vi "MAG_UI_Main_old.vi"() -> ()   [LabVIEW 2016]
doc: "Use this template to build a simple state machine design pattern. Each state executes code and determines which state to transition to."
uses:
  controls/MAG_UI_Data.ctl
  controls/MAG_UI_Command.ctl
  controls/MAG_Comms_State.ctl
  controls/Sensor_Data.ctl
  <vilib>/Math Plots/3D Math Plots/3D Surface/3D Surface XCtrl/3D Surface.xctl
  <vilib>/Math Plots/3D Math Plots/3D Surface/3D Surface Datatype/3D Surface Datatype.lvclass
  controls/MAG_UI_State.ctl
  controls/MAG_Display_State.ctl
  controls/MAG_UI_Comms_Config.ctl
  <vilib>/Math Plots/3D Math Plots/3D Surface/3D Surface Datatype/Public/Plot Helper (Matrix).vi
panel:
  in  "UI_Tab":enum32{"Display", "Config", "Debug"}(tab)
  out "Sensor Readings":dbl[][](array[numeric])=[[53.321, -3127.915, -23851.52], [-458.11, -296.645, -18895.36], [1342.037, -322.179, -20134.399999999998], [1022.111, -1906.789, -22302.72], [2748.66, -1244.407, -21063.68], [-84.112, -4542.048, -19824.64], [307.91, 878.67, -19824.64], [-4568.333, -4041.882, -21373.44], [-6.008, -325.183, -24161.28], [-1336.78, 741.988, -16417.28], [596.294, -402.536, -21373.44], [-4497.739, -1861.729, -15488.0], [-2729.134, -3046.807, -17966.079999999998], [-4886.757, -3190.248, -15488.0], [-5275.775, -1495.241, -18585.6], [-744.241, -4708.019, -20753.92], [-2035.961, 1997.66, -22612.48], [-624.081, -1578.602, -21373.44], [-5331.349, -177.987, -15797.76], [-5163.876, -1893.271, -17656.32], [-6317.412, 26.285, -17036.8], [-5709.853, -1238.3990000000001, -17346.559999999998], [-6253.577, -2501.581, -17346.559999999998], [-4917.548, 525.7, -19514.88], [4038.127, 854.638, -17656.32], [2519.605, -2692.335, -17346.559999999998], [422.062, -178.738, -27878.399999999998], [2497.826, 931.24, -16417.28], [2088.531, 18.024, -17656.32], [-2016.435, -340.954, -16107.52], [1248.162, -1542.554, -20444.16], [-2485.059, -2575.179, -20444.16], [-69.092, -449.098, -22612.48], [-2240.984, 1145.275, -17346.559999999998], [3456.102, 2005.17, -17346.559999999998], [-3088.112, 773.53, -17036.8], [-1416.386, 1058.91, -18585.6], [-1229.387, 273.364, -18895.36], [-4542.048, -1396.86, -18895.36], [-4826.677, -60.08, -16417.28], [1227.134, 4367.065, -21063.68], [1716.786, 2915.382, -20134.399999999998], [-1334.527, 4276.194, -21373.44], [-884.678, 2008.174, -17036.8], [-1700.264, 2225.964, -21063.68], [-1527.534, 1893.271, -18895.36], [-2355.136, 772.028, -17346.559999999998], [-4691.497, -1109.227, -23541.76], [1372.828, 0.0, -23851.52], [-2353.634, 566.254, -21373.44], [-4619.401, 7687.987, -16417.28], [-6183.734, 823.096, -17036.8], [-5976.458, -100.634, -20444.16], [-3851.128, -639.101, -16417.28], [-4383.587, -1360.812, -19205.12], [-3419.303, -80.357, -17966.079999999998], [-3107.638, 4759.838, -22922.239999999998], [-3023.526, 2978.466, -19824.64], [-2249.245, 102.136, -20134.399999999998], [-714.201, -5060.989, -28188.16], [-950.015, 5369.65, -25710.079999999998], [-5348.622, 5862.306, -22612.48], [-3420.054, 3359.223, -19824.64], [-5260.004, 1431.406, -24780.8]]
  in  "Zero":bool
  in  "Tab Control":enum32{"2D", "3D"}(tab)=enum."3D"
  out "Node Response":T1(graph)={"Node XYZ List[0]"=53.321, "Node XYZ List[1]"=-3127.915, "Node XYZ List[2]"=-23851.52}
  in  "Node":i32
  out "3D Surface":refnum<class "3D Plot Datatype.lvclass">[](xcontrol)
  in  "Comms Setting":enum32{"Serial", "Bluetooth"}(tab)
  in  "VISA resource name":refnum<visa-resource-name>="COM16"
  in  "Serial Settings":T2={"baud rate"=57600, "data bits"=8, "parity"=enum."None", "stop bits"=10, "flow control"=0} {"flow control" items=["None"=0, "XON/XOFF"=1, "RTS/CTS"=2, "DTR/DSR"=4]; "stop bits" items=["1.0"=10, "1.5"=15, "2.0"=20]; "data bits" min=5 max=8 step=1; "baud rate" items=["75"=75, "110"=110, "134"=134, "150"=150, "300"=300, "600"=600, "1200"=1200, "1800"=1800, "2400"=2400, "4800"=4800, "7200"=7200, "9600"=9600, "14400"=14400, "19200"=19200, "28800"=28800, "38400"=38400, "56000"=56000, "57600"=57600, "115200"=115200, "128000"=128000, "230400"=230400]}
  out "Comm State":T3
  out "notification":T5
  out "comms":i32=4022
  out "ui":i32=2010
  out "Bytes_In_Buffer":u32
  in  "Button_Disconnect":bool
  in  "Button_Initialise":bool
  in  "Button_Stream":bool
  out "Status":T6={"System Version"="", "Connected"=TRUE, "Active?"=FALSE, "Streaming"=TRUE, "Logging"=FALSE}
  in  "Button_Record":bool
  in  "Button_Sys_Check":bool
  in  "Button_Connect":bool
  in  "Button_Exit":bool
  # "MagBoard n64"
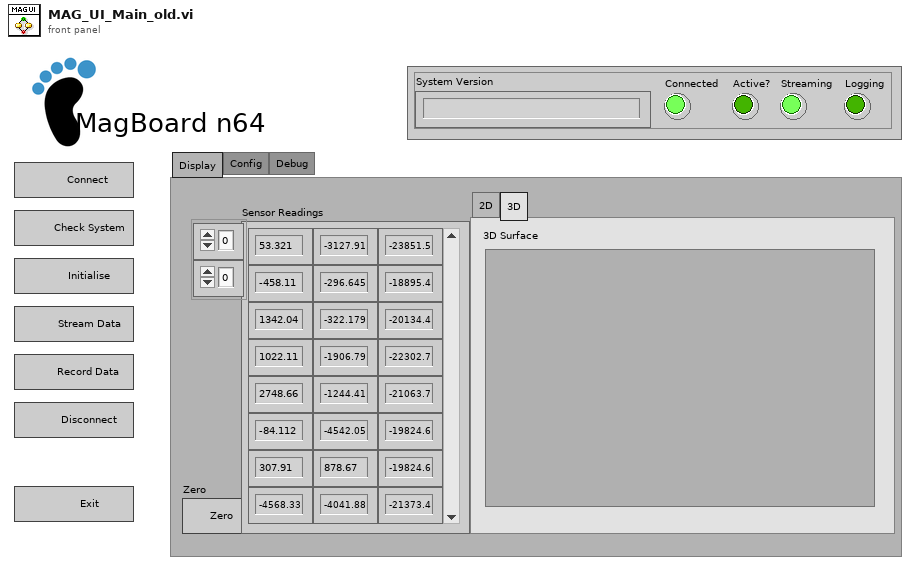
[diagram p1: front panel]
types:
  T1 = cluster{"Node XYZ List[0]":dbl, "Node XYZ List[1]":dbl, "Node XYZ List[2]":dbl}
  T2 = cluster{"baud rate":u32, "data bits":u16, "parity":enum16{"None", "Odd", "Even", "Mark", "Space"}, "stop bits":u16, "flow control":u16}
  T3 = typedef "MAG_UI_Command.ctl" = cluster{"Comms_States":T4, "Parameters":string, "Clear Buffer?":bool}
  T4 = typedef "MAG_Comms_State.ctl" = enum16{"Initialize", "Wait for Event", "Connect", "Send_Com", "Rcv_TXT", "Rcv_BIN", "Rcv_FILE", "Disconnect"}
  T5 = typedef "Sensor_Data.ctl" = cluster{"Time":u32, "Data":i16[]}
  T6 = typedef "MAG_UI_Data.ctl" = cluster{"System Version":string, "Connected":bool, "Active?":bool, "Streaming":bool, "Logging":bool}
  T7 = typedef "MAG_UI_Comms_Config.ctl" = cluster{enum16{"Serial", "Bluetooth"}, "Serial Refnum":refnum<visa-resource-name>}
  T8 = typedef "MAG_Display_State.ctl" = enum16{"Initialise", "Display", "Exit"}
  T9 = typedef "MAG_UI_State.ctl" = enum16{"Initialize", "Wait for Event", "Com_Connect", "Com_Init_Sys", "Com_Chk_Sys", "Com_Stream", "Com_Log", "Exit"}
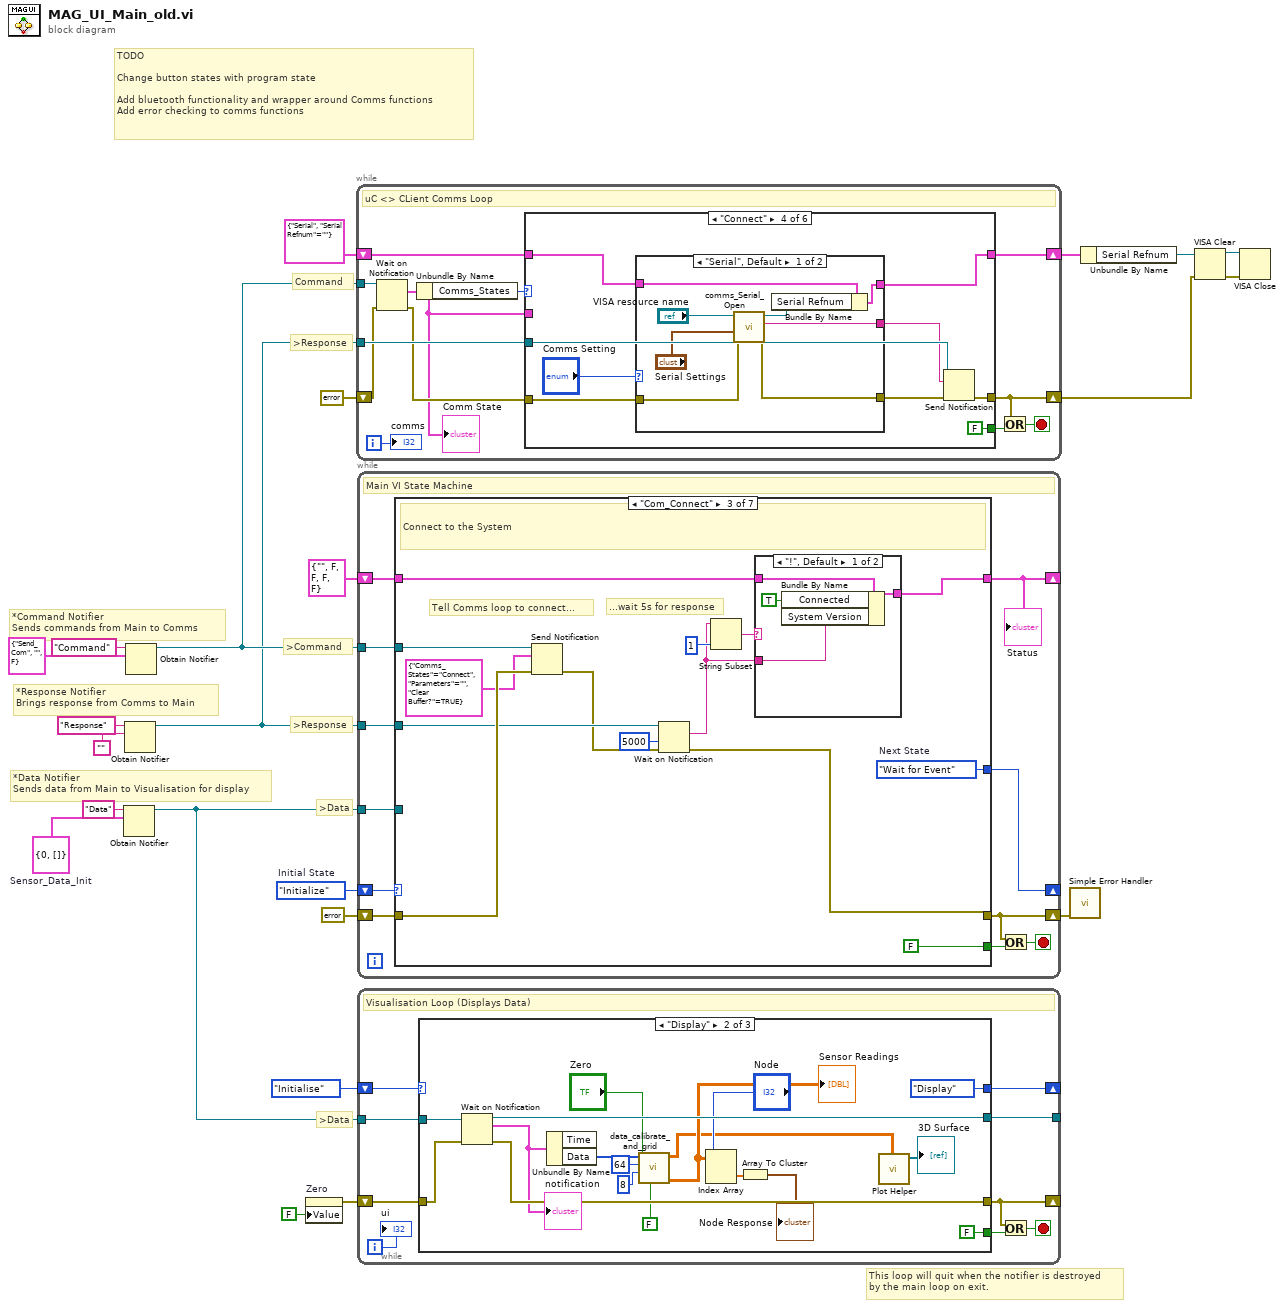
[diagram p0: block diagram]
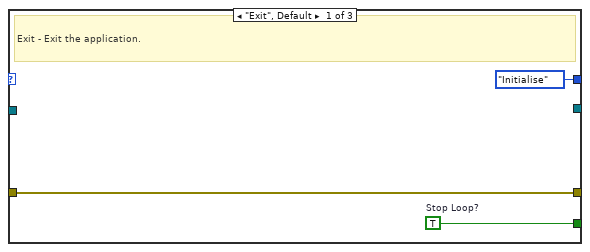
[diagram p2: hidden frame]
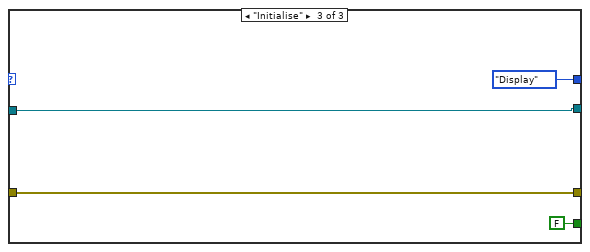
[diagram p3: hidden frame]
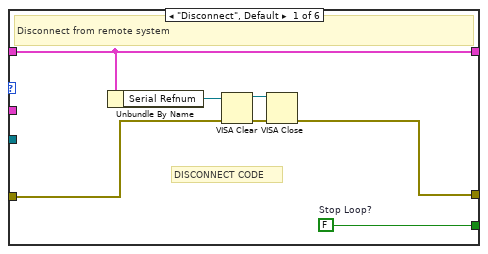
[diagram p4: hidden frame]
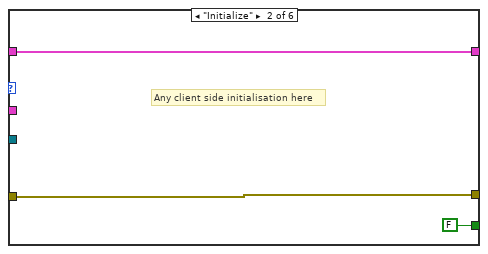
[diagram p5: hidden frame]
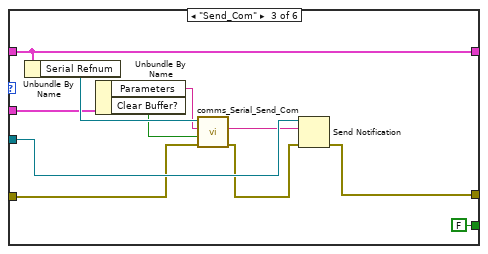
[diagram p6: hidden frame]
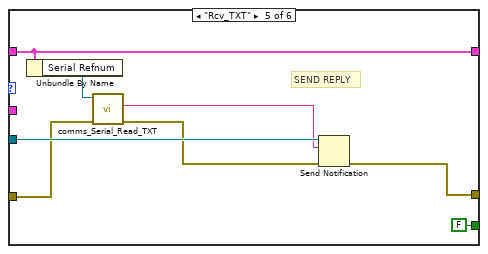
[diagram p8: hidden frame]
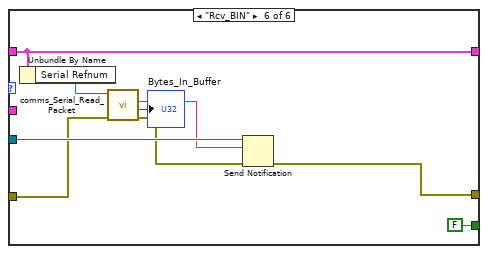
[diagram p9: hidden frame]
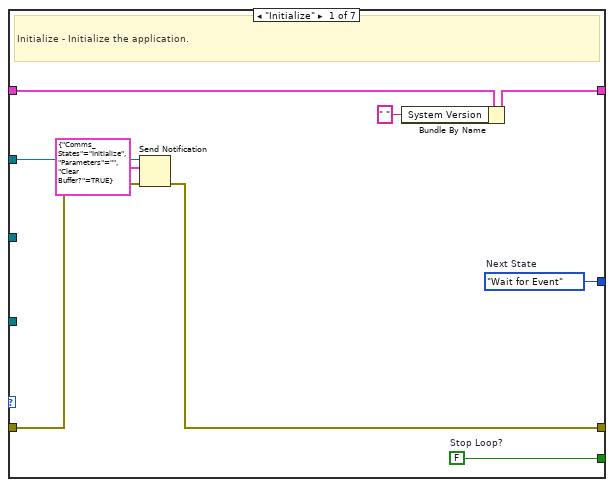
[diagram p10: hidden frame]
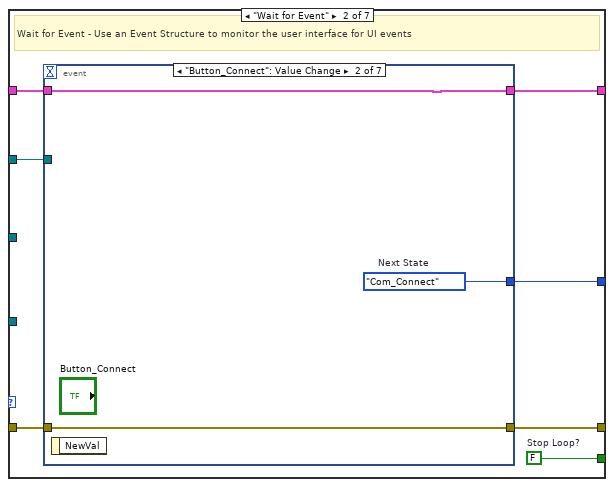
[diagram p11: hidden frame]
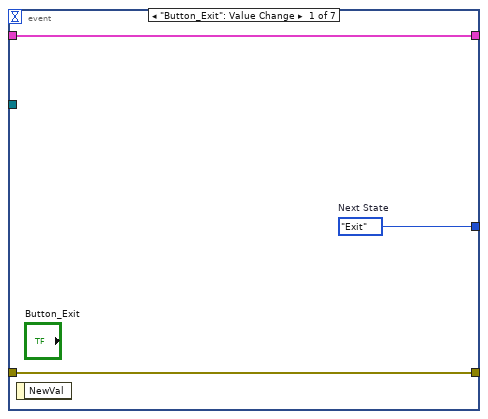
[diagram p12: hidden frame]
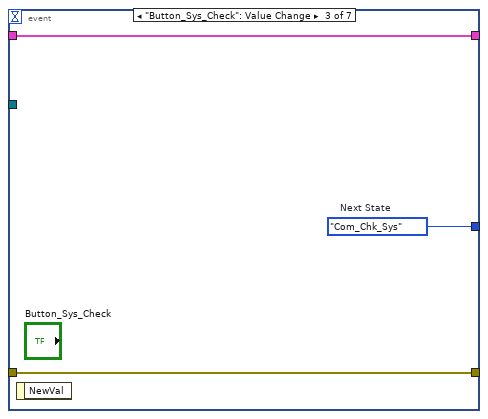
[diagram p13: hidden frame]
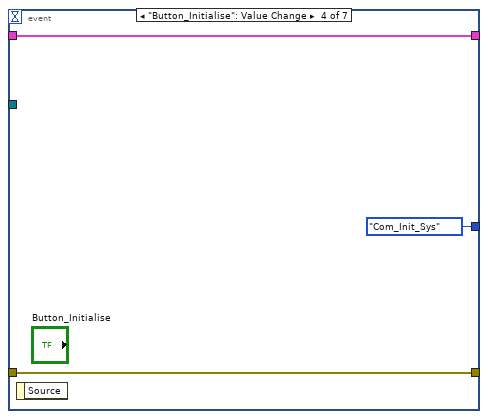
[diagram p14: hidden frame]
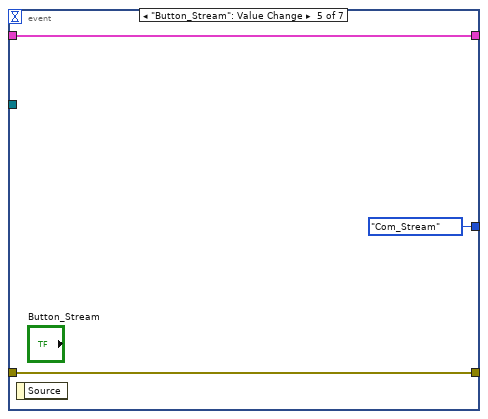
[diagram p15: hidden frame]
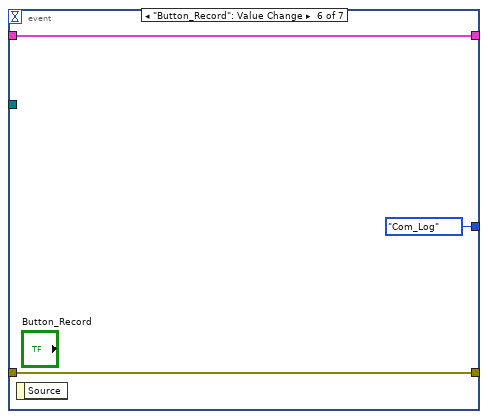
[diagram p16: hidden frame]
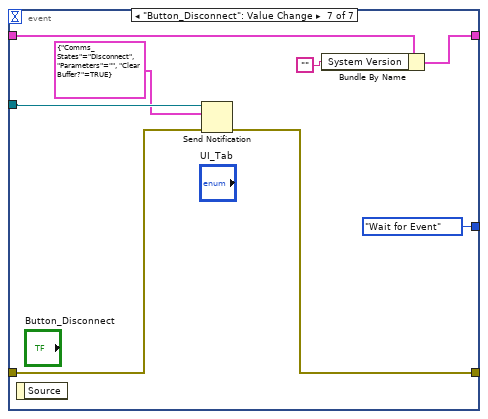
[diagram p17: hidden frame]
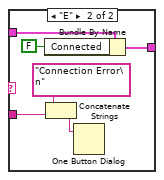
[diagram p18: hidden frame]
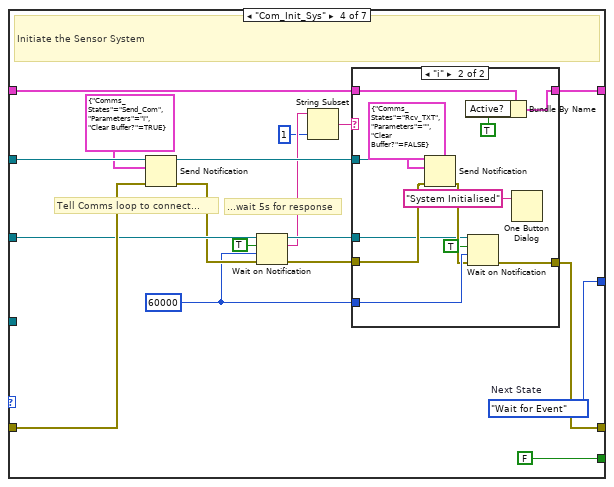
[diagram p19: hidden frame]
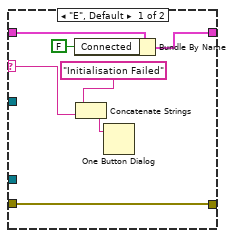
[diagram p20: hidden frame]
diagram:
  w12 = T5 {"Time"=0, "Data"=[]}  # Sensor_Data_Init
  w23 = MAG_UI_State."Initialize"  # Initial State
  # "TODO\n\nChange button states with program state\n\nAdd bluetooth functionality and wrapper around Comms functions\nAdd error checking to comms functions"
  # "This loop will quit when the notifier is destroyed\nby the main loop on exit."
  # ">Data"
  # ">Data"
  # ">Response"
  # ">Response"
  # ">Command"
  # "*Data Notifier\nSends data from Main to Visualisation for display"
  # "*Response Notifier\nBrings response from Comms to Main"
  # "*Command Notifier\nSends commands from Main to Comms"
  # "Command"
  n1 = Obtain Notifier(name (unnamed)="Data", notification data type=w12) -> (notifier out=w14:refnum<notifier>)  [unwired: 2 in, 2 out]
  n2 = Obtain Notifier(name (unnamed)="Response", notification data type="") -> (notifier out=w13:refnum<notifier>)  [unwired: 2 in, 2 out]
  n3 = Obtain Notifier(name (unnamed)="Command", notification data type=T3 {"Comms_States"=enum."Send_Com", "Parameters"="", "Clear Buffer?"=FALSE}) -> (notifier out=w17:refnum<notifier>)  [unwired: 2 in, 2 out]
  n4 = property on="Zero" class="Bool (strict)"("Value"=FALSE ("Zero")) -> (error out=w1:errorcluster)  [unwired: 2 in, 1 out]
  n5 = while {
    shift-right: [w32] -> w3
    shift-left: errorcluster {"status"=FALSE, "code"=0, "source"=""} ("error constant") -> [w29]
    tunnel: w17 -> [w31]
    tunnel: w13 -> [w33]
    shift-right: [w26] -> w4
    shift-left: T7 {enum."Serial", "Serial Refnum"=""} -> [w27]
    i -> [w25]
    stop <- w34 stop-if-true
    # "uC <> CLient Comms Loop"
    n6 = Wait on Notification(notifier=w31, error in (no error)=w29) -> (notification=w24:T3, error out=w28:errorcluster)  [unwired: 2 in, 2 out]
    "Comm State" <- w24
    n7 = Unbundle By Name(w24) -> ("Comms_States"=w30:T4)
    n8 = case shown="\"Connect\"" w30 {
      tunnel: [w42 FALSE ("Stop Loop?") FALSE ("Stop Loop?") FALSE ("Stop Loop?") FALSE ("Stop Loop?") FALSE ("Stop Loop?")] -> w35
      tunnel: w28 -> [w38 w44 w50 w58 w78 w86]
      tunnel: [w37 w44 w55 w65 w82 w91] -> w32
      tunnel: w33 -> [_ _ w56 w62 w83 w90]
      tunnel: w27 -> [w36 w43 w51 w60 w80 w87]
      tunnel: [w36 w43 w51 w59 w80 w87] -> w26
      tunnel: w24 -> [_ _ w47 _ _ _]
      frame "Disconnect", Default {
        w42 = FALSE  # Stop Loop?
        # "DISCONNECT CODE"
        # "Disconnect from remote system"
        n9 = Unbundle By Name(w36) -> ("Serial Refnum"=w41:refnum<visa-resource-name>)
        n10 = VISA Clear(VISA resource name=w41, error in (no error)=w38) -> (VISA resource name out=w39:refnum<visa-resource-name>, error out=w40:errorcluster)
        n11 = VISA Close(VISA resource name=w39, error in (no error)=w40) -> (error out=w37:errorcluster)
      }
      frame "Initialize" {
        # "Any client side initialisation here"
      }
      frame "Send_Com" {
        n12 = Unbundle By Name(w51) -> ("Serial Refnum"=w53:refnum<visa-resource-name>)
        n13 = Unbundle By Name(w47) -> ("Parameters"=w46:string, "Clear Buffer?"=w48:bool)
        n14 = call "comms_Serial_Send_Com.vi"("error in"=w50, "Buffer Clear?"=w48, "Command"=w46, "VISA resource in"=w53) -> ("error out"=w49:errorcluster, "Response"=w52:string)  [unwired: 5 in, 1 out]
        n15 = Send Notification(notification=w52, notifier=w56, error in (no error)=w49) -> (error out=w55:errorcluster)  [unwired: 1 out]
      }
      frame "Connect" {
        n16 = case shown="\"Serial\", Default" "Comms Setting" {
          tunnel: [w67 w74] -> w61
          tunnel: w60 -> [w71 w75]
          tunnel: [w69 w75] -> w59
          tunnel: w58 -> [w68 w74]
          tunnel: [w66 _] -> w57
          frame "Serial", Default {
            n17 = call "comms_Serial_Open.vi"("error in (no error)"=w68, "Serial Settings in"="Serial Settings", "VISA Refnum in"="VISA resource name") -> ("error out"=w67:errorcluster, "Data Out"=w66:string, "VISA Refnum out"=w70:refnum<visa-resource-name>)  [unwired: 6 in]
            n18 = Bundle By Name(cluster=w71, "Serial Refnum"=w70) -> (w69:T7)
          }
          frame "Bluetooth" {
          }
        }
        n19 = Send Notification(notification=w57, notifier=w62, error in (no error)=w61) -> (error out=w65:errorcluster)  [unwired: 1 out]
      }
      frame "Rcv_TXT" {
        # "SEND REPLY"
        n20 = Unbundle By Name(w80) -> ("Serial Refnum"=w79:refnum<visa-resource-name>)
        n21 = call "comms_Serial_Read_TXT.vi"("error in"=w78, "VISA resource in"=w79) -> ("error out"=w77:errorcluster, "Data Out"=w76:string)  [unwired: 6 in, 2 out]
        n22 = Send Notification(notification=w76, notifier=w83, error in (no error)=w77) -> (error out=w82:errorcluster)  [unwired: 1 out]
      }
      frame "Rcv_BIN" {
        n23 = Unbundle By Name(w87) -> ("Serial Refnum"=w88:refnum<visa-resource-name>)
        n24 = call "comms_Serial_Read_Packet.vi"("error in"=w86, "VISA resource in"=w88) -> ("error out"=w85:errorcluster, "Bytes_In_Buffer"=→"Bytes_In_Buffer":u32, "Data Out"=w89:string)  [unwired: 6 in, 1 out]
        n25 = Send Notification(notification=w89, notifier=w90, error in (no error)=w85) -> (error out=w91:errorcluster)  [unwired: 1 out]
      }
    }
    n26 = Or(x=w32, y=w35) -> (x .or. y?=w34:bool)
    "comms" <- w25
  }
  n27 = while {
    shift-right: [w102] -> _
    shift-left: w23 -> [w103]
    shift-right: [w93] -> _
    shift-left: T6 {"System Version"="", "Connected"=FALSE, "Active?"=FALSE, "Streaming"=FALSE, "Logging"=FALSE} ("Data") -> [w101]
    shift-right: [w97] -> w20
    shift-left: errorcluster {"status"=FALSE, "code"=0, "source"=""} ("error constant") -> [w100]
    tunnel: w17 -> [w96]
    tunnel: w13 -> [w95]
    tunnel: w14 -> [w94]
    stop <- w98 stop-if-true
    # "Main VI State Machine"
    n28 = case shown="\"Com_Connect\"" w103 {
      tunnel: [w112 w119 w159 w178 w215 w251 w287] -> w102
      tunnel: [w111 w118 FALSE ("Stop Loop?") FALSE ("Stop Loop?") FALSE ("Stop Loop?") FALSE ("Stop Loop?") w285] -> w99
      tunnel: w101 -> [w110 w117 w151 w182 w219 w255 w286]
      tunnel: [w109 w116 w150 w181 w218 w254 w286] -> w93
      tunnel: w100 -> [w105 w115 w156 w185 w222 w258 w281]
      tunnel: [w104 w114 w153 w175 w212 w248 w280] -> w97
      tunnel: w96 -> [w107 w113 w157 w186 w223 w259 w284]
      tunnel: w95 -> [_ _ w155 w184 w221 w257 w278]
      tunnel: w94 -> [_ _ _ _ _ w244 w277]
      frame "Initialize" {
        w111 = FALSE  # Stop Loop?
        w112 = MAG_UI_State."Wait for Event"  # Next State
        # "Initialize - Initialize the application."
        n29 = Send Notification(notification=T3 {"Comms_States"=enum."Initialize", "Parameters"="", "Clear Buffer?"=TRUE}, notifier=w107, error in (no error)=w105) -> (error out=w104:errorcluster)  [unwired: 1 out]
        n30 = Bundle By Name(cluster=w110, "System Version"=" ") -> (w109:T6)
      }
      frame "Wait for Event" {
        w118 = FALSE  # Stop Loop?
        # "Wait for Event - Use an Event Structure to monitor the user interface for UI events"
        n31 = event shown="[1] \"Button_Connect\": Value Change" {
          selector: _ -> [_ _ _ _ _ _ _]
          dyn-events: _ -> [_ _ _ _ _ _ _]
          timeout: _ -> [_ _ _ _ _ _ _]
          tunnel: [w122 w125 w128 MAG_UI_State."Com_Init_Sys" ("Next State") MAG_UI_State."Com_Stream" ("Next State") MAG_UI_State."Com_Log" ("Next State") MAG_UI_State."Wait for Event" ("Next State")] -> w119
          tunnel: w117 -> [w121 w123 w126 w131 w134 w137 w140]
          tunnel: [w121 w123 w126 w131 w134 w137 w139] -> w116
          tunnel: w115 -> [w120 w124 w127 w130 w133 w136 w143]
          tunnel: [w120 w124 w127 w130 w133 w136 w142] -> w114
          tunnel: w113 -> [_ _ _ _ _ _ w144]
          event "Button_Exit": Value Change {
            w122 = MAG_UI_State."Exit"  # Next State
            n32 = event-data() -> ()  [unwired: 1 in, 1 out]
          }
          event "Button_Connect": Value Change {
            w125 = MAG_UI_State."Com_Connect"  # Next State
            n33 = event-data() -> ()  [unwired: 1 in, 1 out]
          }
          event "Button_Sys_Check": Value Change {
            w128 = MAG_UI_State."Com_Chk_Sys"  # Next State
            n34 = event-data() -> ()  [unwired: 1 in, 1 out]
          }
          event "Button_Initialise": Value Change {
            n35 = event-data() -> ()  [unwired: 1 in, 1 out]
          }
          event "Button_Stream": Value Change {
            n36 = event-data() -> ()  [unwired: 1 in, 1 out]
          }
          event "Button_Record": Value Change {
            n37 = event-data() -> ()  [unwired: 1 in, 1 out]
          }
          event "Button_Disconnect": Value Change {
            n38 = event-data() -> ()  [unwired: 1 in, 1 out]
            n39 = Send Notification(notification=T3 {"Comms_States"=enum."Disconnect", "Parameters"="", "Clear Buffer?"=TRUE}, notifier=w144, error in (no error)=w143) -> (error out=w142:errorcluster)  [unwired: 1 out]
            n40 = Bundle By Name(cluster=w140, "System Version"="") -> (w139:T6)
          }
        }
      }
      frame "Com_Connect" {
        w159 = MAG_UI_State."Wait for Event"  # Next State
        # "...wait 5s for response"
        # "Tell Comms loop to connect..."
        # "Connect to the System"
        n41 = Send Notification(notification=T3 {"Comms_States"=enum."Connect", "Parameters"="", "Clear Buffer?"=TRUE}, notifier=w157, error in (no error)=w156) -> (error out=w154:errorcluster)  [unwired: 1 out]
        n42 = Wait on Notification(notifier=w155, timeout in ms (-1)=5000, error in (no error)=w154) -> (notification=w146:string, error out=w153:errorcluster)  [unwired: 1 in, 2 out]
        n43 = String Subset(string=w146, length (rest)=1 ("offset (0)")) -> (substring=w148:string)  [unwired: 1 in]
        n44 = case shown="\"!\", Default" w148 {
          tunnel: w151 -> [w163 w167]
          tunnel: [w162 w166] -> w150
          tunnel: w146 -> [w160 w164]
          frame "!", Default {
            n45 = Bundle By Name(cluster=w163, "Connected"=TRUE, "System Version"=w160) -> (w162:T6)
          }
          frame "E" {
            n46 = Bundle By Name(cluster=w167, "Connected"=FALSE) -> (w166:T6)
            n47 = Concatenate Strings("Connection Error\n", w164) -> (w169:string)
            n48 = One Button Dialog(message=w169) -> ()  [unwired: 1 in, 1 out]
          }
        }
      }
      frame "Com_Init_Sys" {
        w178 = MAG_UI_State."Wait for Event"  # Next State
        w177 = 60000 ("timeout in ms (-1)")
        # "...wait 5s for response"
        # "Tell Comms loop to connect..."
        # "Initiate the Sensor System"
        n49 = Send Notification(notification=T3 {"Comms_States"=enum."Send_Com", "Parameters"="I", "Clear Buffer?"=TRUE}, notifier=w186, error in (no error)=w185) -> (notifier out=w179:refnum<notifier>, error out=w183:errorcluster)
        n50 = Wait on Notification(notifier=w184, ignore previous (F)=TRUE, timeout in ms (-1)=w177, error in (no error)=w183) -> (notifier out=w174:refnum<notifier>, notification=w171:string, error out=w176:errorcluster)  [unwired: 1 out]
        n51 = String Subset(string=w171, length (rest)=1 ("offset (0)")) -> (substring=w172:string)  [unwired: 1 in]
        n52 = case shown="\"i\"" w172 {
          selector: w172 -> [w192 _]
          tunnel: w182 -> [w191 w198]
          tunnel: [w190 w197] -> w181
          tunnel: w179 -> [_ w205]
          tunnel: w177 -> [_ w204]
          tunnel: w176 -> [w188 w203]
          tunnel: [w188 w201] -> w175
          tunnel: w174 -> [_ w200]
          frame "E", Default {
            n53 = Bundle By Name(cluster=w191, "Connected"=FALSE) -> (w190:T6)
            n54 = Concatenate Strings("Initialisation Failed", w192) -> (w194:string)
            n55 = One Button Dialog(message=w194) -> ()  [unwired: 1 in, 1 out]
          }
          frame "i" {
            n56 = Send Notification(notification=T3 {"Comms_States"=enum."Rcv_TXT", "Parameters"="", "Clear Buffer?"=FALSE}, notifier=w205, error in (no error)=w203) -> (error out=w202:errorcluster)  [unwired: 1 out]
            n57 = Bundle By Name(cluster=w198, "Active?"=TRUE) -> (w197:T6)
            n58 = Wait on Notification(notifier=w200, ignore previous (F)=TRUE, timeout in ms (-1)=w204, error in (no error)=w202) -> (error out=w201:errorcluster)  [unwired: 3 out]
            n59 = One Button Dialog(message="System Initialised") -> ()  [unwired: 1 in, 1 out]
          }
        }
      }
      frame "Com_Chk_Sys" {
        w215 = MAG_UI_State."Wait for Event"  # Next State
        w214 = 5000 ("timeout in ms (-1)")
        # "...wait 5s for response"
        # "Tell Comms loop to connect..."
        # "Check the System Status"
        n60 = Send Notification(notification=T3 {"Comms_States"=enum."Send_Com", "Parameters"="C", "Clear Buffer?"=TRUE}, notifier=w223, error in (no error)=w222) -> (notifier out=w216:refnum<notifier>, error out=w220:errorcluster)
        n61 = Wait on Notification(notifier=w221, ignore previous (F)=TRUE, timeout in ms (-1)=w214, error in (no error)=w220) -> (notifier out=w211:refnum<notifier>, notification=w208:string, error out=w213:errorcluster)  [unwired: 1 out]
        n62 = String Subset(string=w208, length (rest)=1 ("offset (0)")) -> (substring=w209:string)  [unwired: 1 in]
        n63 = case shown="\"c\"" w209 {
          selector: w209 -> [w229 _]
          tunnel: w219 -> [w228 w241]
          tunnel: [w227 w241] -> w218
          tunnel: w216 -> [_ w239]
          tunnel: w214 -> [_ w238]
          tunnel: w213 -> [w225 w237]
          tunnel: [w225 w235] -> w212
          tunnel: w211 -> [_ w234]
          frame "E", Default {
            n64 = Bundle By Name(cluster=w228, "Connected"=FALSE) -> (w227:T6)
            n65 = Concatenate Strings("Initialisation Failed", w229) -> (w231:string)
            n66 = One Button Dialog(message=w231) -> ()  [unwired: 1 in, 1 out]
          }
          frame "c" {
            n67 = Send Notification(notification=T3 {"Comms_States"=enum."Rcv_TXT", "Parameters"="", "Clear Buffer?"=FALSE}, notifier=w239, error in (no error)=w237) -> (error out=w236:errorcluster)  [unwired: 1 out]
            n68 = Wait on Notification(notifier=w234, ignore previous (F)=TRUE, timeout in ms (-1)=w238, error in (no error)=w236) -> (notification=w233:string, error out=w235:errorcluster)  [unwired: 2 out]
            n69 = One Button Dialog(message=w233) -> ()  [unwired: 1 in, 1 out]
          }
        }
      }
      frame "Com_Stream" {
        w251 = MAG_UI_State."Wait for Event"  # Next State
        w250 = 60000 ("timeout in ms (-1)")
        # "...wait 5s for response"
        # "Tell Comms loop to connect..."
        # "Check the System Status"
        n70 = Send Notification(notification=T3 {"Comms_States"=enum."Send_Com", "Parameters"="S", "Clear Buffer?"=TRUE}, notifier=w259, error in (no error)=w258) -> (notifier out=w252:refnum<notifier>, error out=w256:errorcluster)
        n71 = Wait on Notification(notifier=w257, ignore previous (F)=TRUE, timeout in ms (-1)=w250, error in (no error)=w256) -> (notifier out=w247:refnum<notifier>, notification=w242:string, error out=w249:errorcluster)  [unwired: 1 out]
        n72 = String Subset(string=w242, length (rest)=1 ("offset (0)")) -> (substring=w245:string)  [unwired: 1 in]
        n73 = case shown="\"s\"" w245 {
          tunnel: w255 -> [w265 w270]
          tunnel: [w264 w268] -> w254
          tunnel: w252 -> [_ w276]
          tunnel: w250 -> [_ w275]
          tunnel: w249 -> [w262 w274]
          tunnel: [w262 w273] -> w248
          tunnel: w247 -> [_ w272]
          tunnel: w244 -> [_ w271]
          tunnel: w242 -> [w261 _]
          frame "E", Default {
            n74 = Bundle By Name(cluster=w265, "Connected"=FALSE) -> (w264:T6)
            n75 = Concatenate Strings("Stream Failed", w261) -> (w267:string)
            n76 = One Button Dialog(message=w267) -> ()  [unwired: 1 in, 1 out]
          }
          frame "s" {
            n77 = Bundle By Name(cluster=w270, "Streaming"=TRUE) -> (w268:T6)
            n78 = call "stream_data.vi"("timeout in ms (-1)"=w275, "error in (no error)"=w274, "Display"=w271, "Response"=w272, "Command"=w276) -> ("error out"=w273:errorcluster)  [unwired: 6 in]
          }
        }
      }
      frame "Exit", Default {
        w279 = FALSE ("force destroy? (F)")
        w285 = TRUE  # Stop Loop?
        w287 = MAG_UI_State."Exit"  # (Value Not Used)
        # "Exit - Exit the application."
        n79 = Release Notifier(notifier=w284, force destroy? (F)=w279, error in (no error)=w281) -> (error out=w283:errorcluster)  [unwired: 2 out]
        n80 = Release Notifier(notifier=w278, force destroy? (F)=w279, error in (no error)=w283) -> (error out=w282:errorcluster)  [unwired: 2 out]
        n81 = Release Notifier(notifier=w277, force destroy? (F)=w279, error in (no error)=w282) -> (error out=w280:errorcluster)  [unwired: 2 out]
      }
    }
    "Status" <- w93
    n82 = Or(x=w97, y=w99) -> (x .or. y?=w98:bool)
  }
  n83 = while {
    shift-right: [w295] -> _
    shift-left: MAG_Display_State."Initialise" -> [w296]
    shift-right: [w291] -> _
    shift-left: w1 -> [w294]
    tunnel: w14 -> [w290]
    tunnel: [w289] -> _
    i -> [w288]
    stop <- w292 stop-if-true
    # "Visualisation Loop (Displays Data)"
    n84 = case shown="\"Display\"" w296 {
      tunnel: [MAG_Display_State."Initialise" MAG_Display_State."Display" MAG_Display_State."Display"] -> w295
      tunnel: [w299 FALSE ("Stop Loop?") FALSE ("Stop Loop?")] -> w293
      tunnel: w294 -> [w298 w314 w321]
      tunnel: [w298 w313 w321] -> w291
      tunnel: w290 -> [_ w315 w318]
      tunnel: [_ w312 w318] -> w289
      frame "Exit", Default {
        w299 = TRUE  # Stop Loop?
        # "Exit - Exit the application."
      }
      frame "Display" {
        n85 = Wait on Notification(notifier=w315, error in (no error)=w314) -> (notifier out=w312:refnum<notifier>, notification=w309:T5, error out=w313:errorcluster)  [unwired: 2 in, 1 out]
        "notification" <- w309
        n86 = Unbundle By Name(w309) -> ("Data"=w308:i16[])  [unwired: 1 out]
        n87 = call "data_calibrate_and_grid.vi"("Reset"=FALSE, "Tare"="Zero", "Row Length"=8, "No. Nodes"=64, "Sensor Readings (PACKET)"=w308) -> ("Node XYZ List"=w304:dbl[][], "Z (GRID)"=w302:dbl[][])  [unwired: 2 in, 3 out]
        "Sensor Readings" <- w304
        n88 = Index Array(array=w304, index (row)="Node") -> (element=w311:dbl[])  [unwired: 1 in]
        n89 = Array To Cluster(array=w311) -> (cluster=→"Node Response":T1)
        n90 = call-poly <vilib>:"Plot Helper.vi"("z matrix"=w302) -> ("3D Plot lvclass Array out"=→"3D Surface":refnum<class "3D Plot Datatype.lvclass">[])  [unwired: 5 in, 5 out]
      }
      frame "Initialise" {
      }
    }
    n91 = Or(x=w291, y=w293) -> (x .or. y?=w292:bool)
    "ui" <- w288
  }
  n92 = call <vilib>:"Simple Error Handler.vi"("error in (no error)"=w20) -> ()  [unwired: 4 in, 5 out]
  n93 = Unbundle By Name(w4) -> ("Serial Refnum"=w5:refnum<visa-resource-name>)
  n94 = VISA Clear(VISA resource name=w5, error in (no error)=w3) -> (VISA resource name out=w7:refnum<visa-resource-name>, error out=w6:errorcluster)
  n95 = VISA Close(VISA resource name=w7, error in (no error)=w6) -> ()  [unwired: 1 out]
